vi "Write Iterations Number.vi"(8 "error in (no error)":errorcluster, 10 "Iterations Number":u16=1, 11 "FWCS_ACS_Iterator in":refnum<class "FWCS_ACS_Iterator.lvclass">) -> (0 "error out":errorcluster, 3 "FWCS_ACS_Iterator out":refnum<class "FWCS_ACS_Iterator.lvclass">)   [LabVIEW 2018, in "FWCS_ACS_Iterator.lvclass"]
uses:
  FWCS_ACS_Iterator.lvclass
  FWCS_ACS_Iterator.lvclass/FWCS_ACS_Iterator.ctl
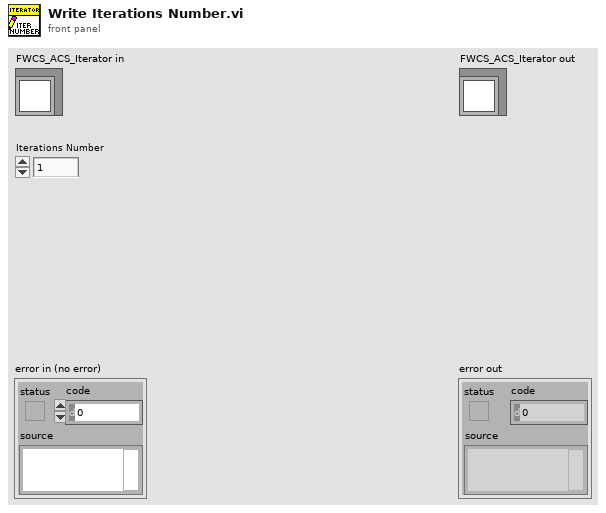
[diagram p1: front panel]
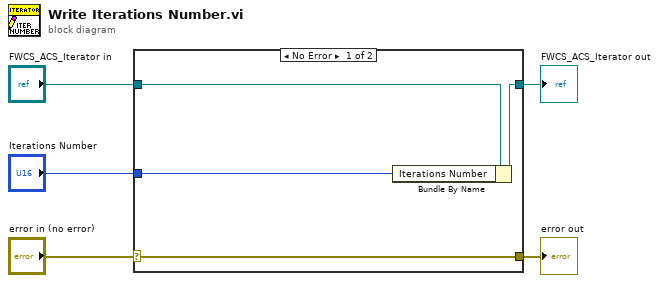
[diagram p0: block diagram]
diagram:
  n1 = case shown="No Error" "error in (no error)" {
    selector: "error in (no error)" -> [w9 w10]
    tunnel: [w9 w10] -> w4
    tunnel: [w7 w11] -> w2
    tunnel: "FWCS_ACS_Iterator in" -> [w8 w11]
    tunnel: "Iterations Number" -> [w6 _]
    frame No Error {
      n2 = Bundle By Name(cluster=w8, "Iterations Number"=w6) -> (w7:refnum<class "FWCS_ACS_Iterator.lvclass">)
    }
    frame Error {
    }
  }
  "error out" <- w4
  "FWCS_ACS_Iterator out" <- w2
